vi "Container.vi"(6 "Start if not running? (T)":bool=TRUE, 7 "Type (inferred)":refnum<class>, 8 "error in (no error)":errorcluster, 10 "Specific":string, 11 "Module Type":refnum<class "RQMHModule.lvclass">) -> (0 "error out":errorcluster, 1 "Handshake (if started)":refnum<class "RQMHStartup.lvclass">, 3 "Module Instance":refnum<class "RQMHModule.lvclass">)   [LabVIEW 2024, in "Module Container.lvlib"]
uses:
  Module Container.lvlib
  Module/RQMHModule.lvclass
  <vilib>/Utility/miscctls.llb/LVMapReplaceAction.ctl
  JQMHStartup/RQMHStartup.lvclass
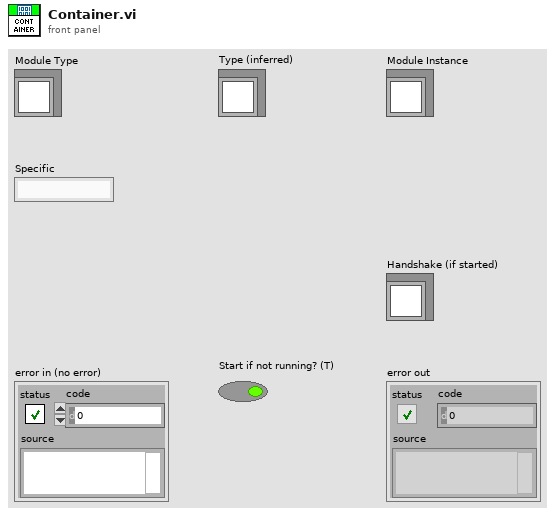
[diagram p1: front panel]
types:
  T1 = typedef "LVMapReplaceAction.ctl" = enum32{"Modify Entry only if found", "Add or Modify Entry", "Delete Entry"}
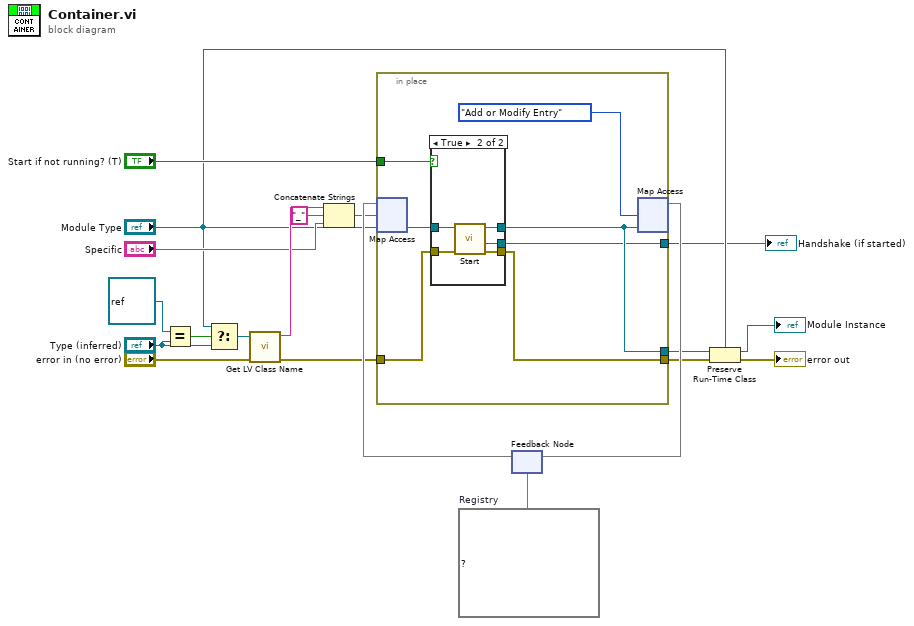
[diagram p0: block diagram]
diagram:
  w20 = map{string, refnum<class "RQMHModule.lvclass">} {}  # Registry
  n1 = Equal?(x=refnum<class> refnum, y="Type (inferred)") -> (x = y?=w14:bool)
  n2 = Select(t="Module Type", s=w14, f="Type (inferred)") -> (s? t:f=w13:refnum<class>)
  n3 = call <vilib>:"Get LV Class Name.vi"("error in (no error)"="error in (no error)", "object"=w13) -> ("error out"=w8:errorcluster, "class name"=w18:string)  [unwired: 8 in]
  n4 = Concatenate Strings(w18, "_" ("string"), "Specific") -> (w10:string)
  n5 = feedback #1(w20) -> (w19:map{string, refnum<class "RQMHModule.lvclass">})
  n6 = in-place {
    in-place-border: w8 -> [w23]
    in-place-border: [w24] -> w3
    in-place-border: [w22] -> w6
    in-place-border: "Start if not running? (T)" -> [w26]
    in-place-border: [w21] -> w1
    n7 = in-place-map #2(w19, w10, "Module Type") -> (w25:refnum<class "RQMHModule.lvclass">)  [unwired: 1 out]
    n8 = case shown="True" w26 {
      tunnel: w25 -> [w29 w34]
      tunnel: w23 -> [w28 w33]
      tunnel: [w28 w32] -> w24
      tunnel: [w29 w31] -> w22
      tunnel: [_ w30] -> w21
      frame False {
      }
      frame True {
        n9 = call "Start.vi"("error in (no error)"=w33, "JQMHCore in"=w34) -> ("error out"=w32:errorcluster, "StartupHandshake out"=w30:refnum<class "RQMHStartup.lvclass">, "JQMHCore out"=w31:refnum<class "RQMHModule.lvclass">)  [unwired: 7 in]
      }
    }
    n10 = in-place-map #2(w22, LVMapReplaceAction."Add or Modify Entry" ("action")) -> (w9:map{string, refnum<class "RQMHModule.lvclass">})  [unwired: 2 out]
  }
  "Handshake (if started)" <- w1
  n11 = feedback-in #1(w9) -> ()
  n12 = Preserve Run-Time Class(object in=w6, error in=w3, 2:"Module Type") -> (object out=→"Module Instance":refnum<class "RQMHModule.lvclass">, error out=→"error out":errorcluster)
